vi "Scan Engine Main Page.vi"(8 "error in (no error)":errorcluster, 11 "Node Ptr":T1 format="%.0x") -> (0 "error out":errorcluster)   [LabVIEW 2017, in "Scan Engine Custom Device.lvlib"]
uses:
  Scan Engine Custom Device.lvlib
  <vilib>/NI Veristand/Custom Device API/Custom Device Item Ref.ctl
  Globals/Property Strings.vi
  <vilib>/NI Veristand/Custom Device API/Get Item Property (U16).vi
  <vilib>/NI Veristand/Custom Device API/Get Item Property (U32).vi
  <vilib>/NI Veristand/Custom Device API/Set Item Property (U32).vi
  <vilib>/NI Veristand/Custom Device API/Set Item Property (U16).vi
  <vilib>/NI Veristand/Custom Device API/Custom Device API.lvlib
panel:
  in  "Delay after FPGA load (s)":u16
  out "Version":string
  in  "SHDocVw.IWebBrowser2":refnum<k7>(container)
  in  "Scan Engine Decimation":u16=1 min=1 max=100
  in  "Sync to Scan?":bool
  in  "Header":cluster{"Section Name":string}={"Section Name"="Scan Engine and EtherCAT Custom Device Settings"}
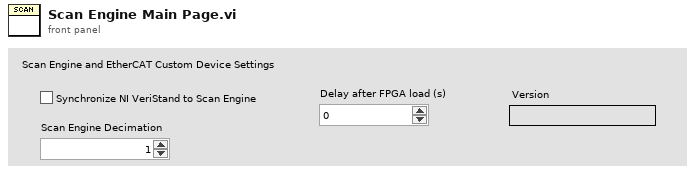
[diagram p1: front panel]
types:
  T1 = typedef "Custom Device API.lvlib/Custom Device Item Ref.ctl" = u64
  T2 = typedef "Custom Device API.lvlib/Custom Device Commands.ctl" = enum16{"Default", "Item renamed", "Shutdown", "Dynamic button pressed"}
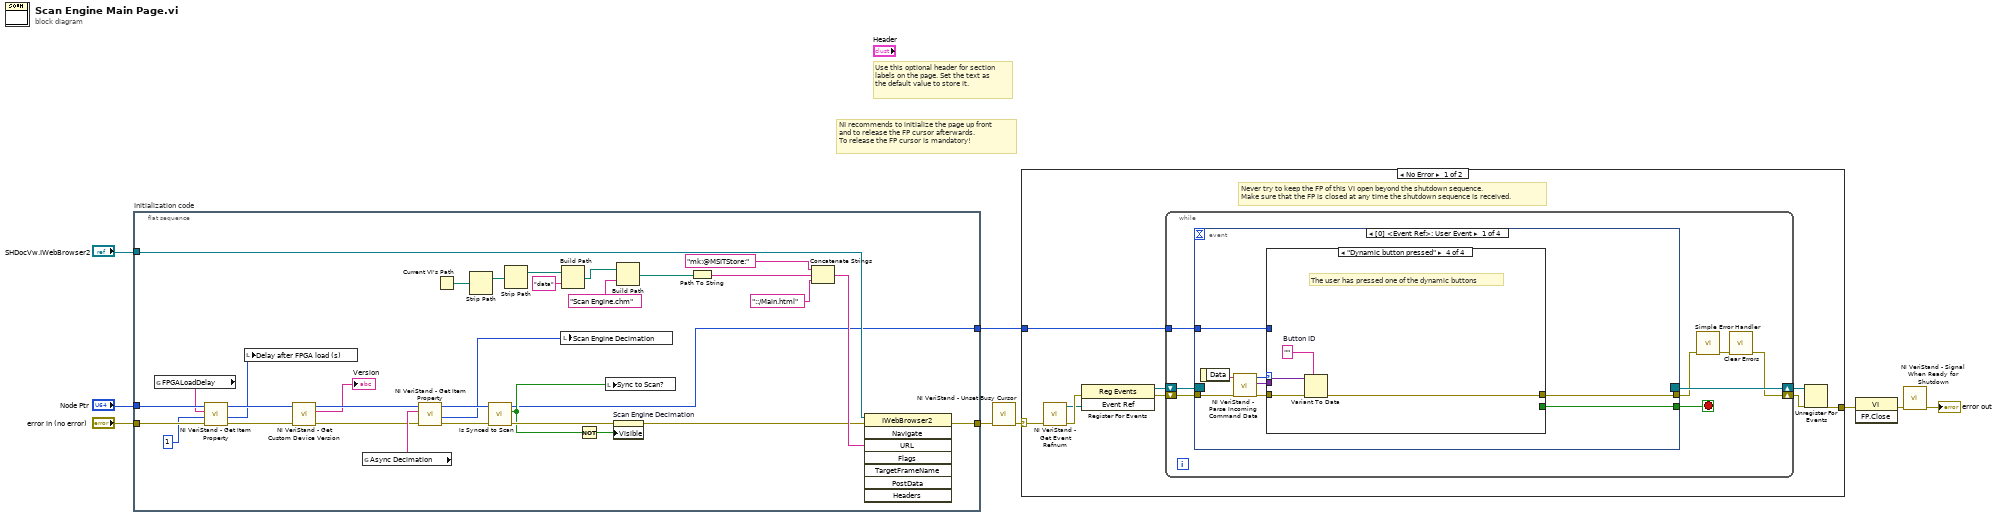
[diagram p0: block diagram]
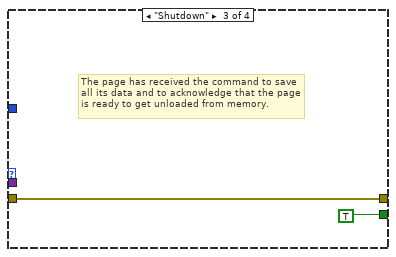
[diagram p4: hidden frame]
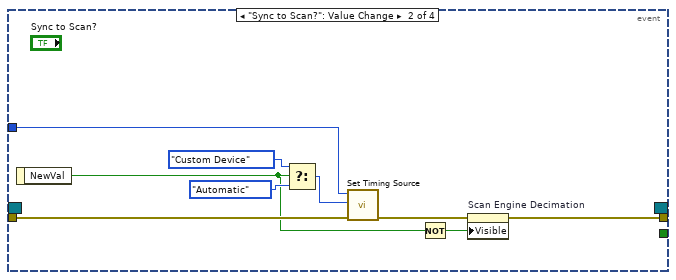
[diagram p5: hidden frame]
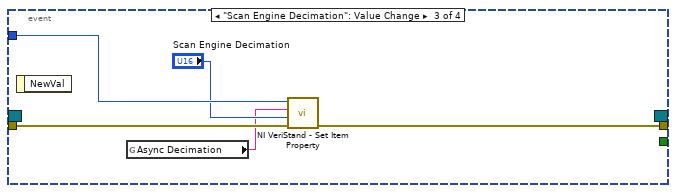
[diagram p6: hidden frame]
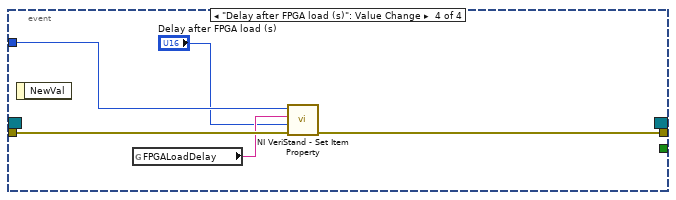
[diagram p7: hidden frame]
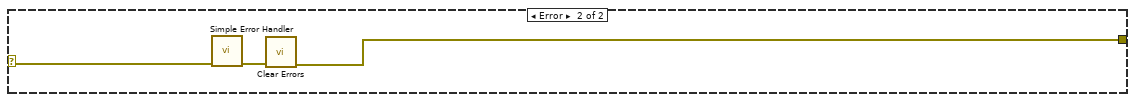
[diagram p8: hidden frame]
diagram:
  # "Use this optional header for section labels on the page. Set the text as the default value to store it."
  # "NI recommends to initialize the page up front\nand to release the FP cursor afterwards.\nTo release the FP cursor is mandatory!"
  n1 = flat-sequence "Initialization code" {
    tunnel: "error in (no error)" -> [w19]
    tunnel: "Node Ptr" -> [w14]
    tunnel: [w34] -> w5
    tunnel: [w20] -> w2
    tunnel: "SHDocVw.IWebBrowser2" -> [w33]
    frame #0 {
      n2 = global read "Property Strings.vi" "FPGALoadDelay"() -> (w11:string)
      n3 = call-poly <vilib>:"NI VeriStand - Get Item Property.vi"("error in (no error)"=w19, "Default Value"=u16 1 ("Delay after FPGA load"), "Property Name"=w11, "Item Ref in"=w14) -> ("error out"=w15:errorcluster, "Value"=w10:u16, "Item Ref out"=w13:T1)  [unwired: 4 in, 1 out]
      n4 = local write "Delay after FPGA load (s)"(w10) -> ()
      n5 = call <vilib>:"NI VeriStand - Get Custom Device Version.vi"("error in (no error)"=w15, "Device Ref in"=w13) -> ("error out"=w18:errorcluster, "Value"=→"Version":string, "Device Ref out"=w17:T1)  [unwired: 7 in]
      n6 = global read "Property Strings.vi" "Async Decimation"() -> (w39:string)
      n7 = call-poly <vilib>:"NI VeriStand - Get Item Property.vi"("error in (no error)"=w18, "Property Name"=w39, "Item Ref in"=w17) -> ("error out"=w41:errorcluster, "Value"=w38:u32, "Item Ref out"=w40:T1)  [unwired: 5 in, 1 out]
      n8 = Current VI's Path() -> (path=w31:path)
      n9 = Strip Path(path=w31) -> (stripped path=w30:path)  [unwired: 1 out]
      n10 = call "Is Synced to Scan.vi"("error in"=w41, "Item Ref in"=w40) -> ("error out"=w37:errorcluster, "Sync to Scan?"=w36:bool, "Item Ref out"=w20:T1)  [unwired: 6 in, 1 out]
      n11 = Strip Path(path=w30) -> (stripped path=w24:path)  [unwired: 1 out]
      n12 = local write "Scan Engine Decimation"(w38) -> ()
      n13 = Build Path(base path=w24, name or relative path="data") -> (appended path=w23:path)
      n14 = Not(x=w36) -> (.not. x?=w35:bool)
      n15 = local write "Sync to Scan?"(w36) -> ()
      n16 = property on="Scan Engine Decimation" class="DigNum (strict)"(error in=w37, "Visible"=w35) -> (error out=w21:errorcluster)  [unwired: 1 in, 1 out]
      n17 = Build Path(base path=w23, name or relative path="Scan Engine.chm") -> (appended path=w27:path)
      n18 = Path To String(path=w27) -> (string=w28:string)
      n19 = Concatenate Strings("mk:@MSITStore:" ("string"), w28, "::/Main.html" ("name or relative path")) -> (w25:string)
      n20 = invoke class="IWebBrowser2" method="Navigate"(reference=w33, error in=w21, "URL"=w25) -> (error out=w34:errorcluster)  [unwired: 5 in, 7 out]
    }
  }
  n21 = call <vilib>:"NI VeriStand - Unset Busy Cursor.vi"("error in (no error)"=w5) -> ("error out"=w4:errorcluster)  [unwired: 10 out]
  n22 = case shown="No Error" w4 {
    selector: w4 -> [w42 w96]
    tunnel: [w47 w94] -> w9
    tunnel: w2 -> [w43 _]
    frame No Error {
      # "Never try to keep the FP of this VI open beyond the shutdown sequence.\nMake sure that the FP is closed at any time the shutdown sequence is received."
      n23 = call <vilib>:"NI VeriStand - Get Event Refnum.vi"("error in (no error)"=w42) -> ("error out"=w50:errorcluster, "Event Ref"=w46:refnum<user-event>)  [unwired: 9 out]
      n24 = register-events(error in=w50, w46) -> (reference out=w44:refnum<event-registration>, error out=w45:errorcluster)  [unwired: 1 in]
      n25 = while {
        tunnel: w43 -> [w54]
        shift-right: [w51] -> w48
        shift-left: w45 -> [w57]
        shift-right: [w58] -> w49
        shift-left: w44 -> [w56]
        stop <- w55 stop-if-true
        n26 = event shown="[0] <Event Ref>: User Event" {
          selector: w56 -> [_ _ _ _]
          dyn-events: [_ _ _ _] -> w58
          timeout: _ -> [_ _ _ _]
          tunnel: w57 -> [w66 w79 w88 w93]
          tunnel: [w62 _ _ _] -> w55
          tunnel: [w61 w76 w87 w92] -> w53
          tunnel: w54 -> [w60 w83 w86 w91]
          event User Event {
            n27 = event-data() -> ("Data"=w65:string)  [unwired: 1 out]
            n28 = call <vilib>:"NI VeriStand - Parse Incoming Command Data.vi"("error in (no error)"=w66, "Incoming data"=w65) -> ("error out"=w64:errorcluster, "Outgoing data"=w59:variant, "Action"=w63:T2)  [unwired: 7 out]
            n29 = case shown="\"Dynamic button pressed\"" w63 {
              tunnel: w64 -> [w67 w68 w69 w74]
              tunnel: [_ _ TRUE _] -> w62
              tunnel: [w67 w68 w69 w71] -> w61
              tunnel: w60 -> [_ _ _ _]
              tunnel: w59 -> [_ _ _ w73]
              frame "Default", Default {
              }
              frame "Item renamed" {
              }
              frame "Shutdown" {
                # "The page has received the command to save all its data and to acknowledge that the page is ready to get unloaded from memory."
              }
              frame "Dynamic button pressed" {
                w72 = ""  # Button ID
                # "The user has pressed one of the dynamic buttons"
                n30 = Variant To Data(error in=w74, type=w72, Variant=w73) -> (error out=w71:errorcluster)  [unwired: 1 out]
              }
            }
          }
          event "Sync to Scan?": Value Change {
            n31 = event-data() -> ("NewVal"=w75:bool)  [unwired: 1 out]
            n32 = Select(t=enum16{"Automatic", "Custom Device"}."Custom Device" ("Timing Source"), s=w75, f=enum16{"Automatic", "Custom Device"}."Automatic" ("Timing Source")) -> (s? t:f=w81:enum16{"Automatic", "Custom Device"})
            n33 = call "Set Timing Source.vi"("error in (no error)"=w79, "Timing Source"=w81, "Item Ref in"=w83) -> ("error out"=w77:errorcluster)  [unwired: 7 in, 1 out]
            n34 = Not(x=w75) -> (.not. x?=w78:bool)
            n35 = property on="Scan Engine Decimation" class="DigNum (strict)"(error in=w77, "Visible"=w78) -> (error out=w76:errorcluster)  [unwired: 1 in, 1 out]
          }
          event "Scan Engine Decimation": Value Change {
            n36 = event-data() -> ()  [unwired: 2 out]
            n37 = global read "Property Strings.vi" "Async Decimation"() -> (w84:string)
            n38 = call-poly <vilib>:"NI VeriStand - Set Item Property.vi"("error in (no error)"=w88, "Value"="Scan Engine Decimation", "Property Name"=w84, "Item Ref in"=w86) -> ("error out"=w87:errorcluster)  [unwired: 5 in, 2 out]
          }
          event "Delay after FPGA load (s)": Value Change {
            n39 = event-data() -> ()  [unwired: 2 out]
            n40 = global read "Property Strings.vi" "FPGALoadDelay"() -> (w90:string)
            n41 = call-poly <vilib>:"NI VeriStand - Set Item Property.vi"("error in (no error)"=w93, "Value"="Delay after FPGA load (s)", "Property Name"=w90, "Item Ref in"=w91) -> ("error out"=w92:errorcluster)  [unwired: 5 in, 2 out]
          }
        }
        n42 = call <vilib>:"Simple Error Handler.vi"("error in (no error)"=w53) -> ("error out"=w52:errorcluster)  [unwired: 1 in, 7 out]
        n43 = call <vilib>:"Clear Errors.vi"("error in (no error)"=w52) -> ("error out"=w51:errorcluster)  [unwired: 1 in, 5 out]
      }
      n44 = Unregister For Events(event registration refnum=w49, error in=w48) -> (error out=w47:errorcluster)
    }
    frame Error {
      n45 = call <vilib>:"Simple Error Handler.vi"("error in (no error)"=w96) -> ("error out"=w95:errorcluster)  [unwired: 1 in, 7 out]
      n46 = call <vilib>:"Clear Errors.vi"("error in (no error)"=w95) -> ("error out"=w94:errorcluster)  [unwired: 1 in, 5 out]
    }
  }
  n47 = invoke class="VI" method="FP.Close"(error in=w9) -> (error out=w8:errorcluster)  [unwired: 2 in, 2 out]
  n48 = call <vilib>:"NI VeriStand - Signal When Ready for Shutdown.vi"("error in (no error)"=w8) -> ("error out"=→"error out":errorcluster)  [unwired: 10 out]
